vi "Append List to Report.vi"(0 "report in":refnum<class "NI_Standard Report.lvclass">, 1 "ordered item type (default)":T1(ring), 2 "unordered item type (default)":enum16{"(default)", "disc", "square", "circle"}(ring), 7 "list elements":string[](array[string]), 9 "list type (ordered)":enum16{"unordered", "ordered"}(ring)=enum."ordered", 11 "error in (no error)":errorcluster, 12 "ordered start (1)":i32=1, 13 "bookmark (Word)":string) -> (4 "report out":refnum<class "NI_Standard Report.lvclass">, 8 "start out (Word)":i32, 10 "end out (Word)":i32, 15 "error out":errorcluster)   [LabVIEW 2015, in "NI_Standard Report.lvclass"]
doc: "Adds a list of elements to the report. If you select <B>ordered</B>, the list is numbered or lettered."
uses:
  <vilib>/Utility/NIReport.llb/Standard Report/NI_Standard Report.lvclass
  <vilib>/Utility/NIReport.llb/Standard Report/NI_Standard Report.lvclass/NI_Standard Report.ctl
  <vilib>/Utility/NIReport.llb/NI_ReportGenerationCore.lvlib
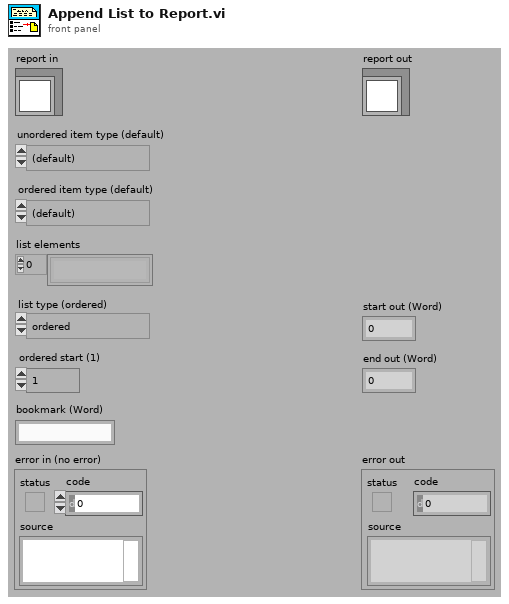
[diagram p1: front panel]
types:
  T1 = enum16{"(default)", "arabic numerals", "lower alpha", "upper alpha"}
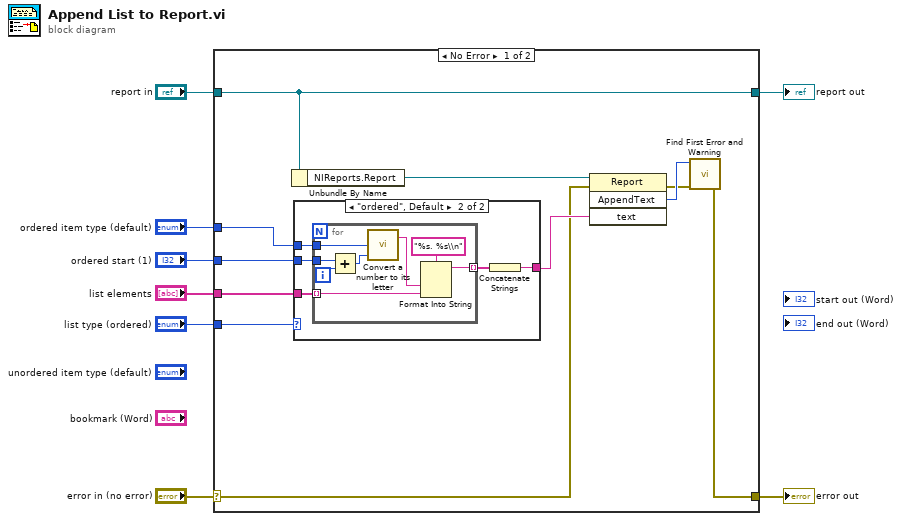
[diagram p0: block diagram]
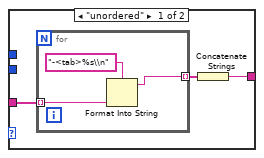
[diagram p2: hidden frame]
diagram:
  n1 = case shown="No Error" "error in (no error)" {
    selector: "error in (no error)" -> [w10 w40]
    tunnel: [w9 w40] -> w7
    tunnel: [w15 w39] -> w5
    tunnel: "report in" -> [w15 w39]
    tunnel: "ordered item type (default)" -> [w14 _]
    tunnel: "ordered start (1)" -> [w13 _]
    tunnel: "list elements" -> [w12 _]
    tunnel: "list type (ordered)" -> [w11 _]
    frame No Error {
      n2 = Unbundle By Name(w15) -> ("NIReports.Report"=w16:refnum<k7>)
      n3 = case shown="\"ordered\", Default" w11 {
        tunnel: w12 -> [w22 w30]
        tunnel: [w20 w28] -> w17
        tunnel: w14 -> [_ w27]
        tunnel: w13 -> [_ w26]
        frame "unordered" {
          n4 = for {
            tunnel: w22 -> [w24] mode=indexing
            tunnel: [w23] -> w21 mode=indexing
            n5 = Format Into String(format string="-<tab>%s\\n", w24) -> (resulting string=w23:string)  [unwired: 2 in, 1 out]
          }
          n6 = Concatenate Strings(w21) -> (w20:string)
        }
        frame "ordered", Default {
          n7 = for {
            tunnel: w30 -> [w36] mode=indexing
            tunnel: [w37] -> w29 mode=indexing
            tunnel: w27 -> [w34]
            tunnel: w26 -> [w31]
            i -> [w33]
            n8 = Add(x=w31, y=w33) -> (x+y=w32:i32)
            n9 = call <vilib>:"Convert a number to its letter.vi"("Number"=w32, "ordered item type (default)"=w34) -> ("string"=w35:string)  [unwired: 2 out]
            n10 = Format Into String(format string="%s. %s\\n", w35, w36) -> (resulting string=w37:string)  [unwired: 2 in, 1 out]
          }
          n11 = Concatenate Strings(w29) -> (w28:string)
        }
      }
      n12 = invoke class="Report" method="AppendText"(reference=w16, error in=w10, "text"=w17) -> (error out=w18:errorcluster, "AppendText"=w19:i32)  [unwired: 1 in, 2 out]
      n13 = call <vilib>:"Find First Error and Warning.vi"("error in (no error)"=w18, "error code"=w19) -> ("error out"=w9:errorcluster)  [unwired: 1 in, 4 out]
    }
    frame Error {
    }
  }
  "error out" <- w7
  "report out" <- w5
